vi "CommonVIs_ColorMemory.vi"(0 "ColorName":variant, 1 "Color In":u32(colorbox), 2 "error in (no error)":errorcluster, 6 "Method (Get Color)":T1) -> (10 "Names":string[](array[string]), 12 "Colors":u32[](array[colorbox]), 14 "Color Out":u32(colorbox), 16 "error out":errorcluster)   [LabVIEW 2020]
doc: "This VI is used to manage system paths.\n\nName: The name of the path to be set or retrieved. The default Name is Home.\n\nPath In: Used to specify the path for Set Path method.\n\nPath Out: Returns the path for Get Path method.\n\nerror out: Returns error info if appropriate.\n\nMethod: {Get Path, Set Path, Delete Path, Clear All Paths}\n\nAuthor: SPCase\nCopyright 2003 VI Engineering, Inc.\n\nCurrent Revision: 12\nVSS Version: 2"
uses:
  <resource>/Framework/Providers/Open_GDS/ClassProviders/Common/CommonVIs/CommonVIs_ColorMemoryAction.ctl
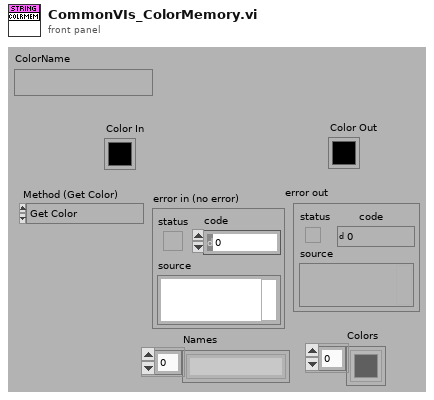
[diagram p1: front panel]
types:
  T1 = typedef "CommonVIs_ColorMemoryAction.ctl" = enum16{"Get Color", "Set Color", "Delete Color", "Clear All Colors"}
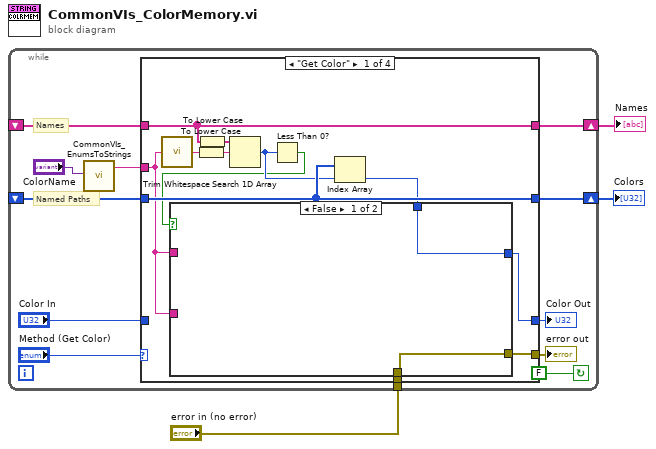
[diagram p0: block diagram]
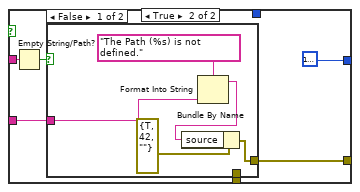
[diagram p2: hidden frame]
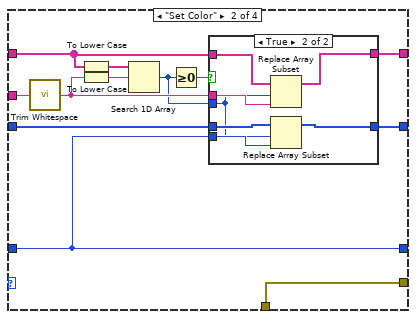
[diagram p4: hidden frame]
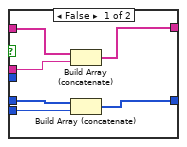
[diagram p5: hidden frame]
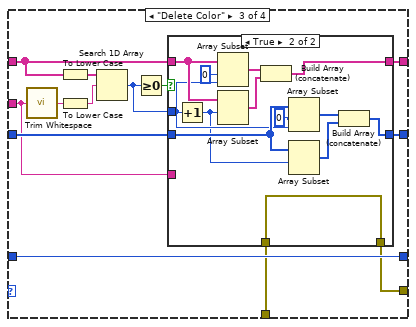
[diagram p6: hidden frame]
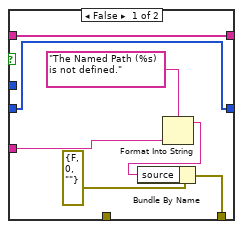
[diagram p7: hidden frame]
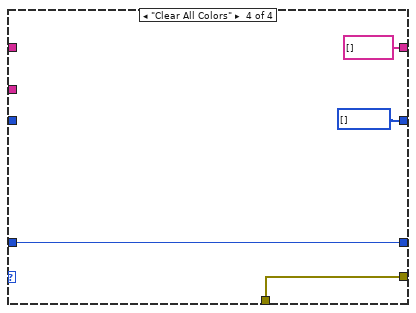
[diagram p8: hidden frame]
diagram:
  n1 = while {
    shift-left: _ -> [w13]
    shift-right: [w12] -> w2
    shift-left: _ -> [w11]
    shift-right: [w10] -> w3
    tunnel: "error in (no error)" -> [w4]
    stop <- FALSE continue-if-true
    # "Named Paths"
    # "Names"
    n2 = call <resource>:"CommonVIs_EnumsToStrings.vi"("SingleEnumVariantIn"="ColorName") -> ("EnumItem"=w5:string)  [unwired: 2 in, 16 out]
    n3 = case shown="\"Get Color\"" "Method (Get Color)" {
      tunnel: "Color In" -> [_ w45 w72 w103]
      tunnel: w5 -> [w17 w53 w70 _]
      tunnel: w13 -> [w21 w51 w79 _]
      tunnel: [w21 w50 w78 string[] []] -> w12
      tunnel: w11 -> [w24 w47 w75 _]
      tunnel: [w24 w46 w74 u32[] []] -> w10
      tunnel: [w26 w45 w72 w103] -> w9
      tunnel: [w27 w42 w71 w100] -> w8
      tunnel: w4 -> [w16 w42 w67 w100]
      frame "Get Color" {
        n4 = call <vilib>:"Trim Whitespace.vi"("string"=w17) -> ("trimmed string"=w25:string)  [unwired: 1 in]
        n5 = To Lower Case(string=w25) -> (all lower case string=w20:string)
        n6 = To Lower Case(string=w21) -> (all lower case string=w19:string[])
        n7 = Search 1D Array(1D array=w19, element=w20) -> (index of element=w23:i32)  [unwired: 1 out]
        n8 = Less Than 0?(x=w23) -> (x < 0?=w18:bool)
        n9 = Index Array(array=w24, index=w23) -> (element=w22:u32)
        n10 = case shown="False" w18 {
          tunnel: [w28 w35] -> w27
          tunnel: [w29 u32 16777216] -> w26
          tunnel: w22 -> [w29 _]
          tunnel: w17 -> [_ w34]
          tunnel: w17 -> [_ w33]
          tunnel: w16 -> [w28 w31]
          frame False {
          }
          frame True {
            n11 = Empty String/Path?(string/path=w33) -> (empty?=w32:bool)
            n12 = case shown="False" w32 {
              tunnel: [w40 w41] -> w35
              tunnel: w34 -> [w36 _]
              tunnel: w31 -> [_ w41]
              frame False {
                n13 = Format Into String(format string="The Path (%s) is not defined.", w36) -> (resulting string=w37:string)  [unwired: 2 in, 1 out]
                n14 = Bundle By Name(cluster=errorcluster {"status"=TRUE, "code"=42, "source"=""} ("error out"), "source"=w37) -> (w40:errorcluster)
              }
              frame True {
              }
            }
          }
        }
      }
      frame "Set Color" {
        n15 = call <vilib>:"Trim Whitespace.vi"("string"=w53) -> ("trimmed string"=w52:string)  [unwired: 1 in]
        n16 = To Lower Case(string=w51) -> (all lower case string=w43:string[])
        n17 = To Lower Case(string=w52) -> (all lower case string=w44:string)
        n18 = Search 1D Array(1D array=w43, element=w44) -> (index of element=w48:i32)  [unwired: 1 out]
        n19 = Greater Or Equal To 0?(x=w48) -> (x >= 0?=w49:bool)
        n20 = case shown="True" w49 {
          tunnel: w52 -> [w58 w66]
          tunnel: w51 -> [w59 w65]
          tunnel: [w57 w64] -> w50
          tunnel: w48 -> [_ w60]
          tunnel: w47 -> [w56 w63]
          tunnel: [w55 w61] -> w46
          tunnel: w45 -> [w54 w62]
          frame False {
            n21 = Build Array (concatenate)(w59, w58) -> (w57:string[])
            n22 = Build Array (concatenate)(w56, w54) -> (w55:u32[])
          }
          frame True {
            n23 = Replace Array Subset(array=w65, new element=w66, index=w60) -> (w64:string[])
            n24 = Replace Array Subset(array=w63, new element=w62, index=w60) -> (w61:u32[])
          }
        }
      }
      frame "Delete Color" {
        n25 = call <vilib>:"Trim Whitespace.vi"("string"=w70) -> ("trimmed string"=w73:string)  [unwired: 1 in]
        n26 = To Lower Case(string=w79) -> (all lower case string=w68:string[])
        n27 = To Lower Case(string=w73) -> (all lower case string=w69:string)
        n28 = Search 1D Array(1D array=w68, element=w69) -> (index of element=w76:i32)  [unwired: 1 out]
        n29 = Greater Or Equal To 0?(x=w76) -> (x >= 0?=w77:bool)
        n30 = case shown="True" w77 {
          tunnel: w79 -> [w86 w99]
          tunnel: [w86 w96] -> w78
          tunnel: w76 -> [_ w90]
          tunnel: w75 -> [w85 w91]
          tunnel: [w85 w88] -> w74
          tunnel: [w80 w87] -> w71
          tunnel: w70 -> [w81 _]
          tunnel: w67 -> [_ w87]
          frame False {
            n31 = Format Into String(format string="The Named Path (%s) is not defined.", w81) -> (resulting string=w84:string)  [unwired: 2 in, 1 out]
            n32 = Bundle By Name(cluster=errorcluster {"status"=FALSE, "code"=0, "source"=""} ("error out"), "source"=w84) -> (w80:errorcluster)
          }
          frame True {
            n33 = Increment(x=w90) -> (x+1=w89:i32)
            n34 = Array Subset(array=w99, index=0, length=w90) -> (w98:string[])
            n35 = Array Subset(array=w99, index=w89) -> (w97:string[])  [unwired: 1 in]
            n36 = Build Array (concatenate)(w98, w97) -> (w96:string[])
            n37 = Array Subset(array=w91, index=0, length=w90) -> (w92:u32[])
            n38 = Array Subset(array=w91, index=w89) -> (w93:u32[])  [unwired: 1 in]
            n39 = Build Array (concatenate)(w92, w93) -> (w88:u32[])
          }
        }
      }
      frame "Clear All Colors" {
      }
    }
    "error out" <- w8
    "Color Out" <- w9
  }
  "Colors" <- w3
  "Names" <- w2
